vi "String To Float_csm.vi"(2 "Default(0)":dbl, 5 "String":string) -> (0 "Float":dbl format="%.2f")   [LabVIEW 2017, in "API String Arguments Support.lvlib"]
uses:
  API String Arguments Support.lvlib
  <userlib>/_NEVSTOP/Communicable State Machine(CSM)/Communicable State Machine.lvlib
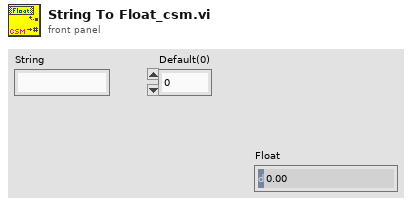
[diagram p1: front panel]
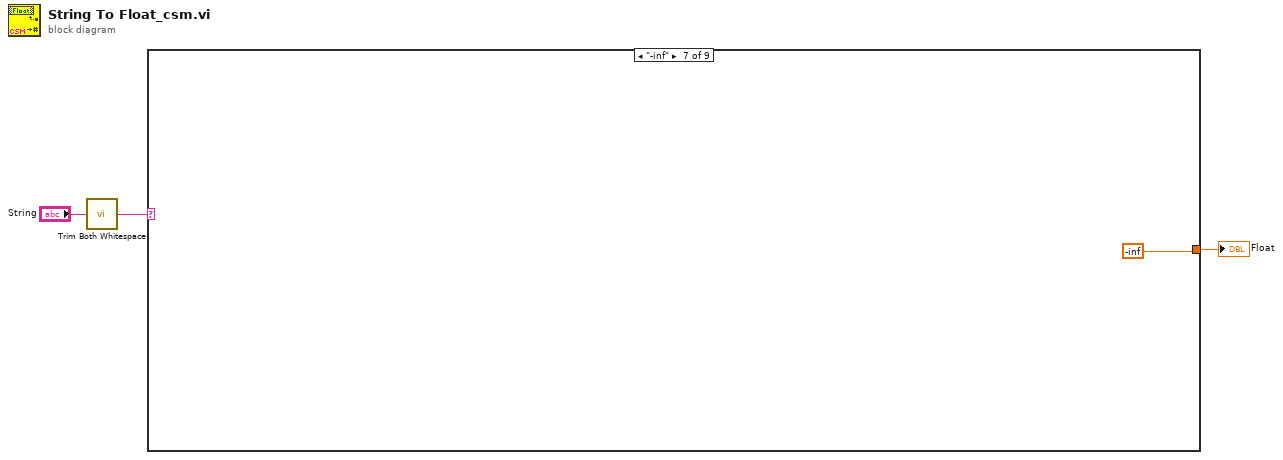
[diagram p0: block diagram]
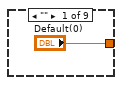
[diagram p2: hidden frame]
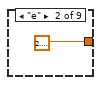
[diagram p3: hidden frame]
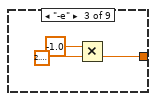
[diagram p4: hidden frame]
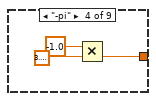
[diagram p5: hidden frame]
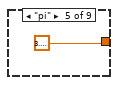
[diagram p6: hidden frame]
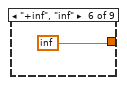
[diagram p7: hidden frame]
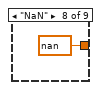
[diagram p8: hidden frame]
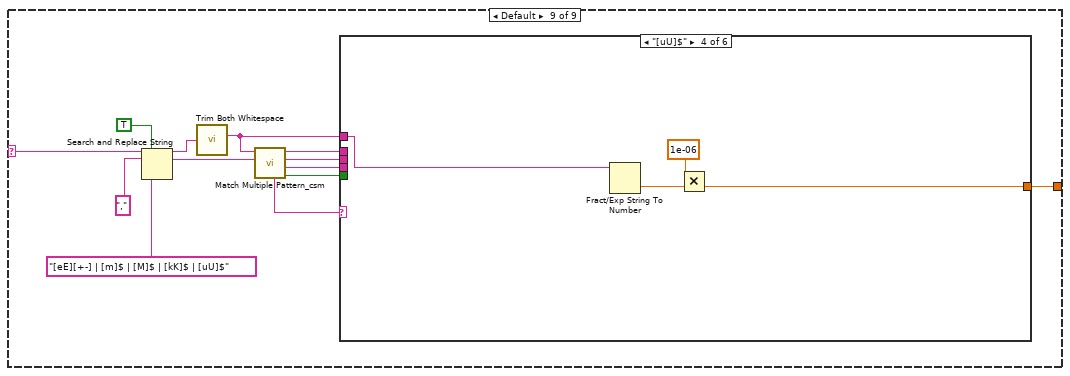
[diagram p9: hidden frame]
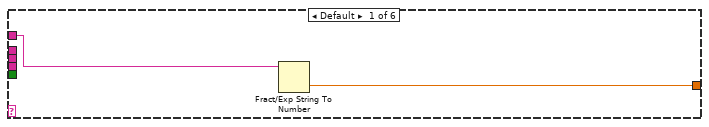
[diagram p10: hidden frame]
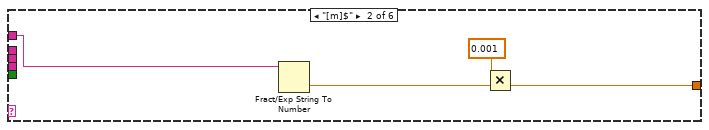
[diagram p11: hidden frame]
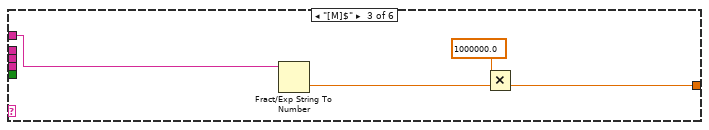
[diagram p12: hidden frame]
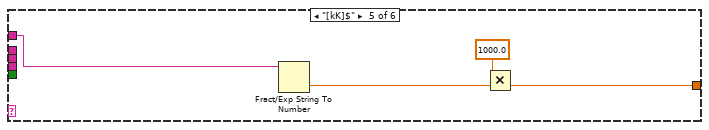
[diagram p13: hidden frame]
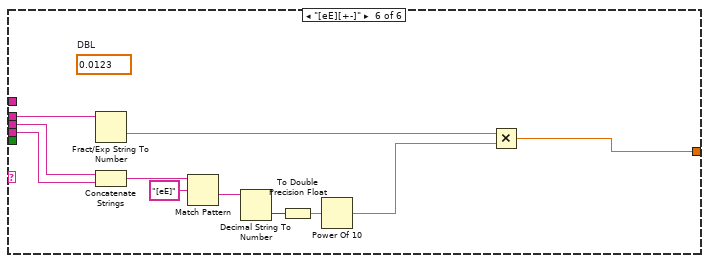
[diagram p14: hidden frame]
diagram:
  n1 = call <userlib>:"Trim Both Whitespace.vi"("string"="String") -> ("trimmed string"=w1:string)  [unwired: 1 in]
  n2 = case shown="\"-inf\"" w1 {
    selector: w1 -> [_ _ _ _ _ _ _ _ w16]
    tunnel: ["Default(0)" 2.718281828459045 w7 w10 3.141592653589793 inf -inf nan ("Default(0)") w19] -> w2
    frame "" {
    }
    frame "e" {
    }
    frame "-e" {
      n3 = Multiply(x=-1.0, y=2.718281828459045) -> (x*y=w7:dbl)
    }
    frame "-pi" {
      n4 = Multiply(x=-1.0, y=3.141592653589793) -> (x*y=w10:dbl)
    }
    frame "pi" {
    }
    frame "+inf", "inf" {
    }
    frame "-inf" {
    }
    frame "NaN" {
    }
    frame Default {
      n5 = Search and Replace String(replace all?=TRUE ("replace all? (F)"), input string=w16, search string=",") -> (result string=w25:string)  [unwired: 5 in, 3 out]
      n6 = call <userlib>:"Trim Both Whitespace.vi"("string"=w25) -> ("trimmed string"=w18:string)  [unwired: 1 in]
      n7 = call "Match Multiple Pattern_csm.vi"("regular expression"="[eE][+-] | [m]$ | [M]$ | [kK]$ | [uU]$", "string"=w18) -> ("Found?"=w23:bool, "after substring"=w21:string, "match substring"=w17:string, "before substring"=w20:string, "pattern matched"=w22:string)  [unwired: 5 in]
      n8 = case shown="\"[uU]$\"" w22 {
        tunnel: w21 -> [_ _ _ _ _ w55]
        tunnel: w20 -> [_ _ _ _ _ w56]
        tunnel: [w28 w31 w35 w39 w43 w46] -> w19
        tunnel: w18 -> [w29 w33 w37 w41 w45 _]
        tunnel: w23 -> [_ _ _ _ _ _]
        tunnel: w17 -> [_ _ _ _ _ w54]
        frame Default {
          n9 = Fract/Exp String To Number(string=w29) -> (number=w28:dbl)  [unwired: 3 in, 1 out]
        }
        frame "[m]$" {
          n10 = Fract/Exp String To Number(string=w33) -> (number=w32:dbl)  [unwired: 3 in, 1 out]
          n11 = Multiply(x=0.001, y=w32) -> (x*y=w31:dbl)
        }
        frame "[M]$" {
          n12 = Fract/Exp String To Number(string=w37) -> (number=w36:dbl)  [unwired: 3 in, 1 out]
          n13 = Multiply(x=1000000.0, y=w36) -> (x*y=w35:dbl)
        }
        frame "[uU]$" {
          n14 = Fract/Exp String To Number(string=w41) -> (number=w40:dbl)  [unwired: 3 in, 1 out]
          n15 = Multiply(x=1e-06, y=w40) -> (x*y=w39:dbl)
        }
        frame "[kK]$" {
          n16 = Fract/Exp String To Number(string=w45) -> (number=w44:dbl)  [unwired: 3 in, 1 out]
          n17 = Multiply(x=1000.0, y=w44) -> (x*y=w43:dbl)
        }
        frame "[eE][+-]" {
          (unwired) 0.0123  # DBL
          n18 = Fract/Exp String To Number(string=w56) -> (number=w48:dbl)  [unwired: 3 in, 1 out]
          n19 = Concatenate Strings(w54, w55) -> (w53:string)
          n20 = Match Pattern(string=w53, regular expression="[eE]") -> (after substring=w51:string)  [unwired: 1 in, 3 out]
          n21 = Decimal String To Number(string=w51) -> (number=w50:i32)  [unwired: 2 in, 1 out]
          n22 = To Double Precision Float(number=w50) -> (double precision float=w49:dbl)
          n23 = Power Of 10(x=w49) -> (10^x=w47:dbl)
          n24 = Multiply(x=w48, y=w47) -> (x*y=w46:dbl)
        }
      }
    }
  }
  "Float" <- w2
